vi "Flux_Capacitor_SoftFP.vi"(0 "reference in":refnum<class "Flux_Capacitor.lvclass">, 2 "Floating":bool, 5 "error in (no error)":errorcluster) -> (14 "reference out":refnum<class "Flux_Capacitor.lvclass">, 19 "error out":errorcluster)   [LabVIEW 2022 SP3, in "Flux_Capacitor.lvlib" / "Flux_Capacitor.lvclass"]
uses:
  Flux_Capacitor.lvclass
  Components/ViPER.lvlibp/ViPER.lvclass
  C:/Projects/Medulla/ViPER/Examples/Flux_Capacitor_Tester/Components/ViPER.lvlibp/ViPER.lvclass
panel:
  in  "Tab Control":enum32{"Flux", "Temp", "Time Circuit"}(tab)
  out "OK":bool
  in  "Flux Test":bool
  out "Temp table":i32(listbox)
  in  "Refresh Temps":bool
  in  "RTC":timestamp format="%<%X\n%x>T"
  in  "Refresh RTC":bool
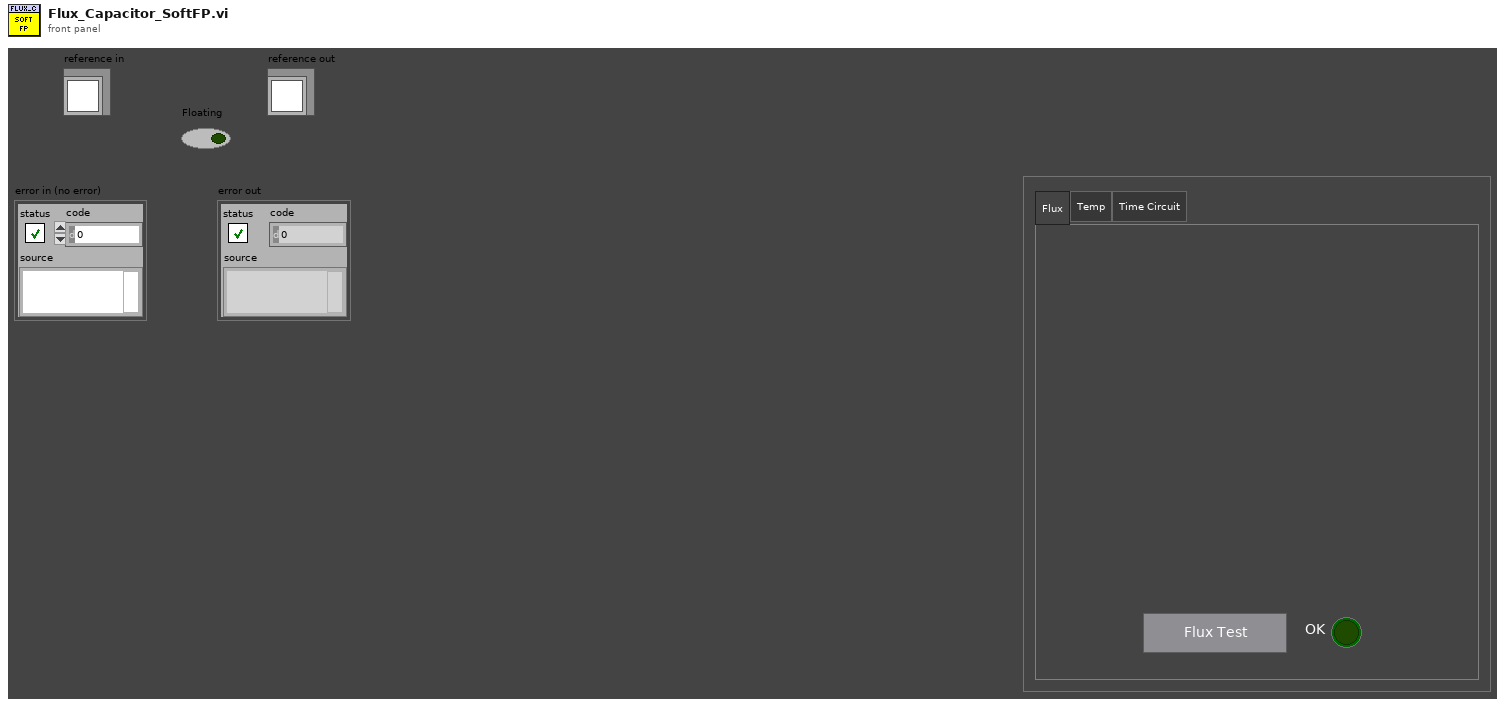
[diagram p1: front panel]
types:
  T1 = enum32{"Invalid", "Standard", "Closed", "Hidden", "Minimized", "Maximized"}
  T2 = typedef "Flux_Capacitor.lvlib/Flux_Capacitor.lvclass/ObjectAttributes.ctl" = cluster{"Config":T3, "T Sensors":T4[], "Temp_DegC":dbl[], "Temp_Raw":u64[], "RTC":timestamp, "Flux":bool, "Time":timestamp, "RTC_Live":timestamp}
  T3 = typedef "Flux_Capacitor.lvlib/Flux_Capacitor.lvclass/Config.ctl" = cluster{"default":string}
  T4 = typedef "Flux_Capacitor.lvlib/Flux_Capacitor.lvclass/TempSensor.ctl" = enum16{"1", "2", "3"}
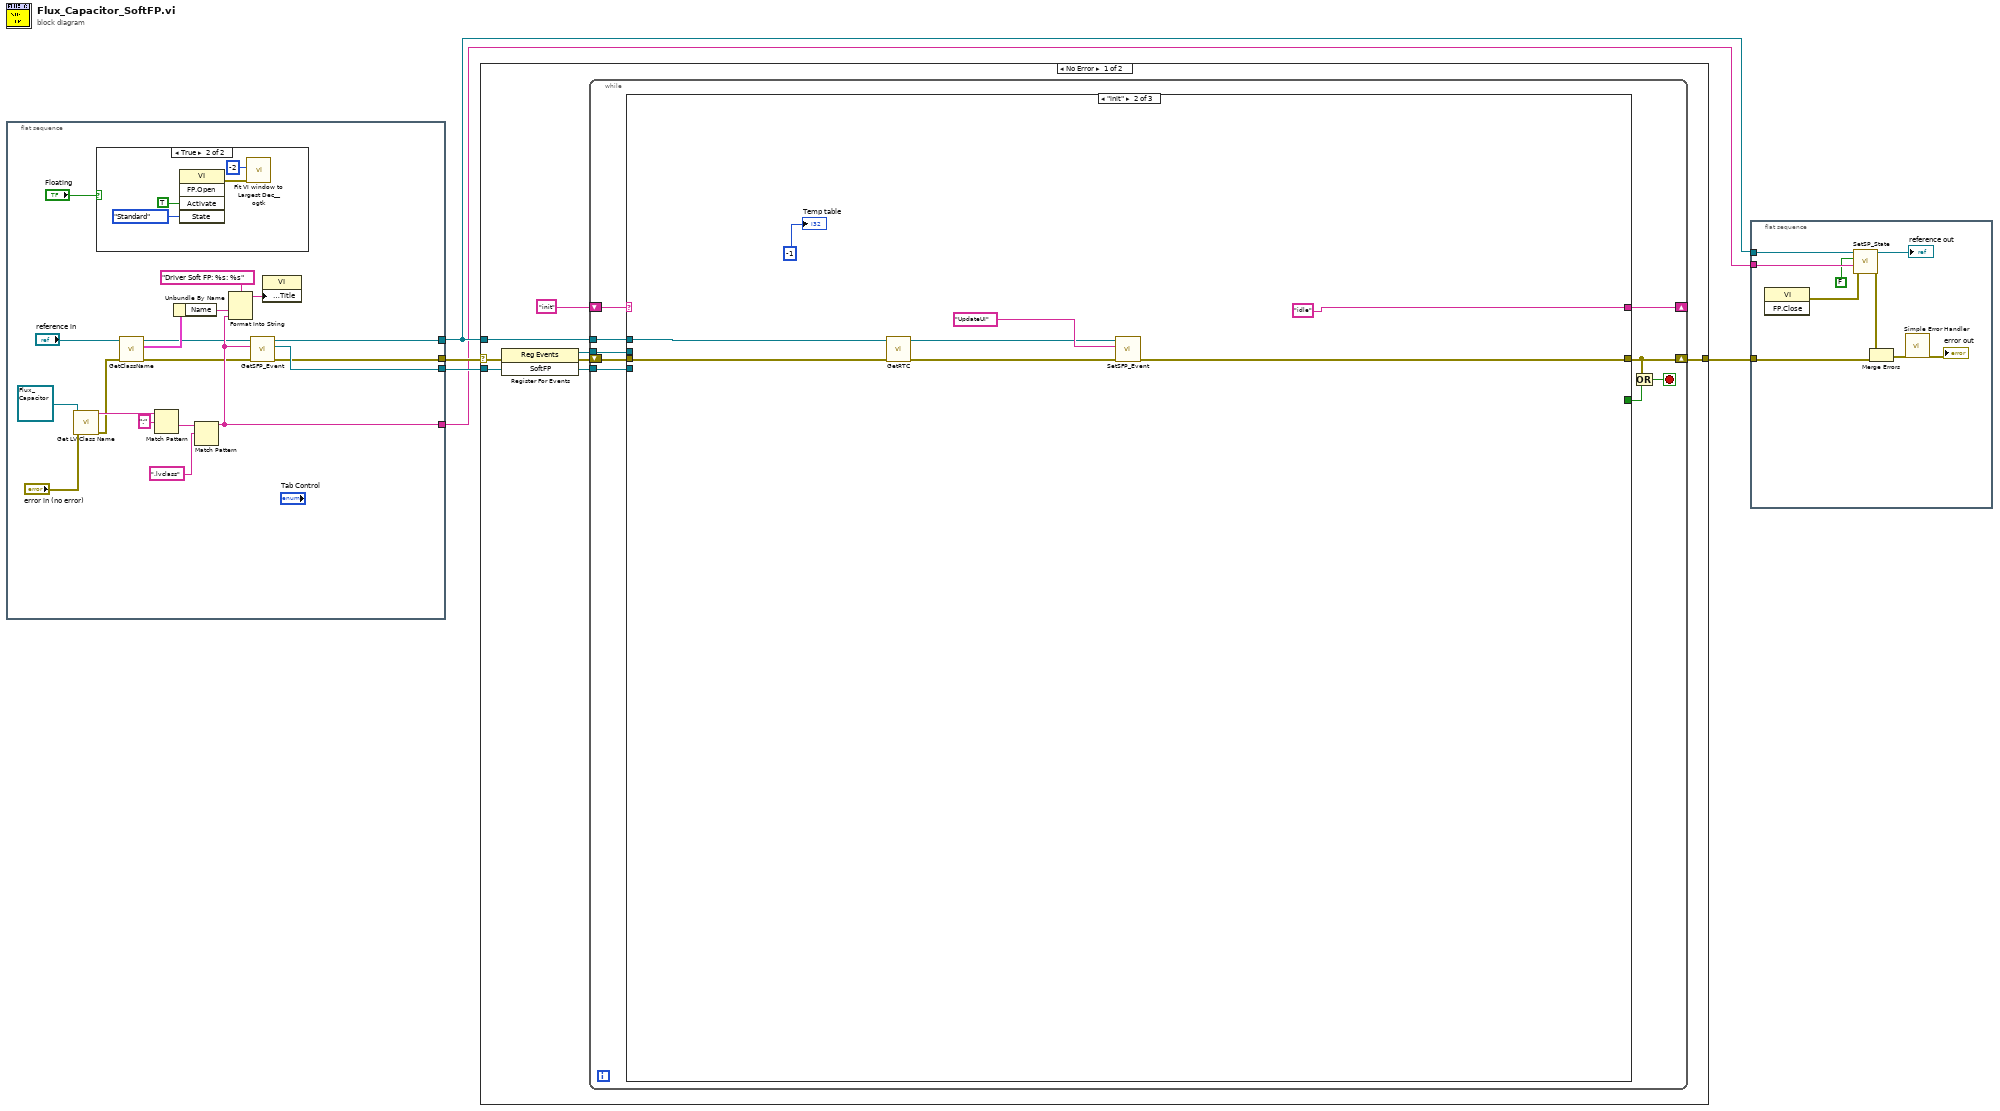
[diagram p0: block diagram]
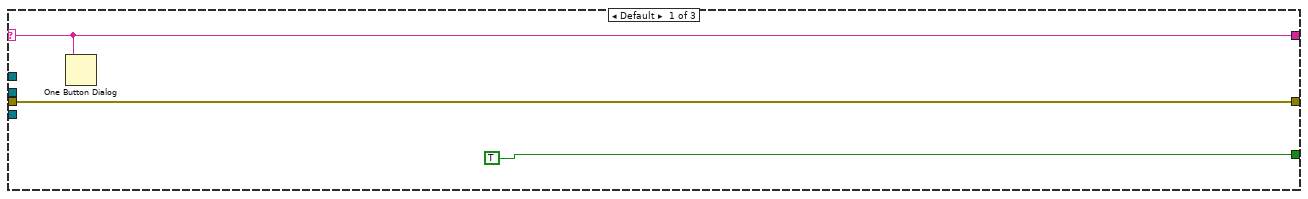
[diagram p3: hidden frame]
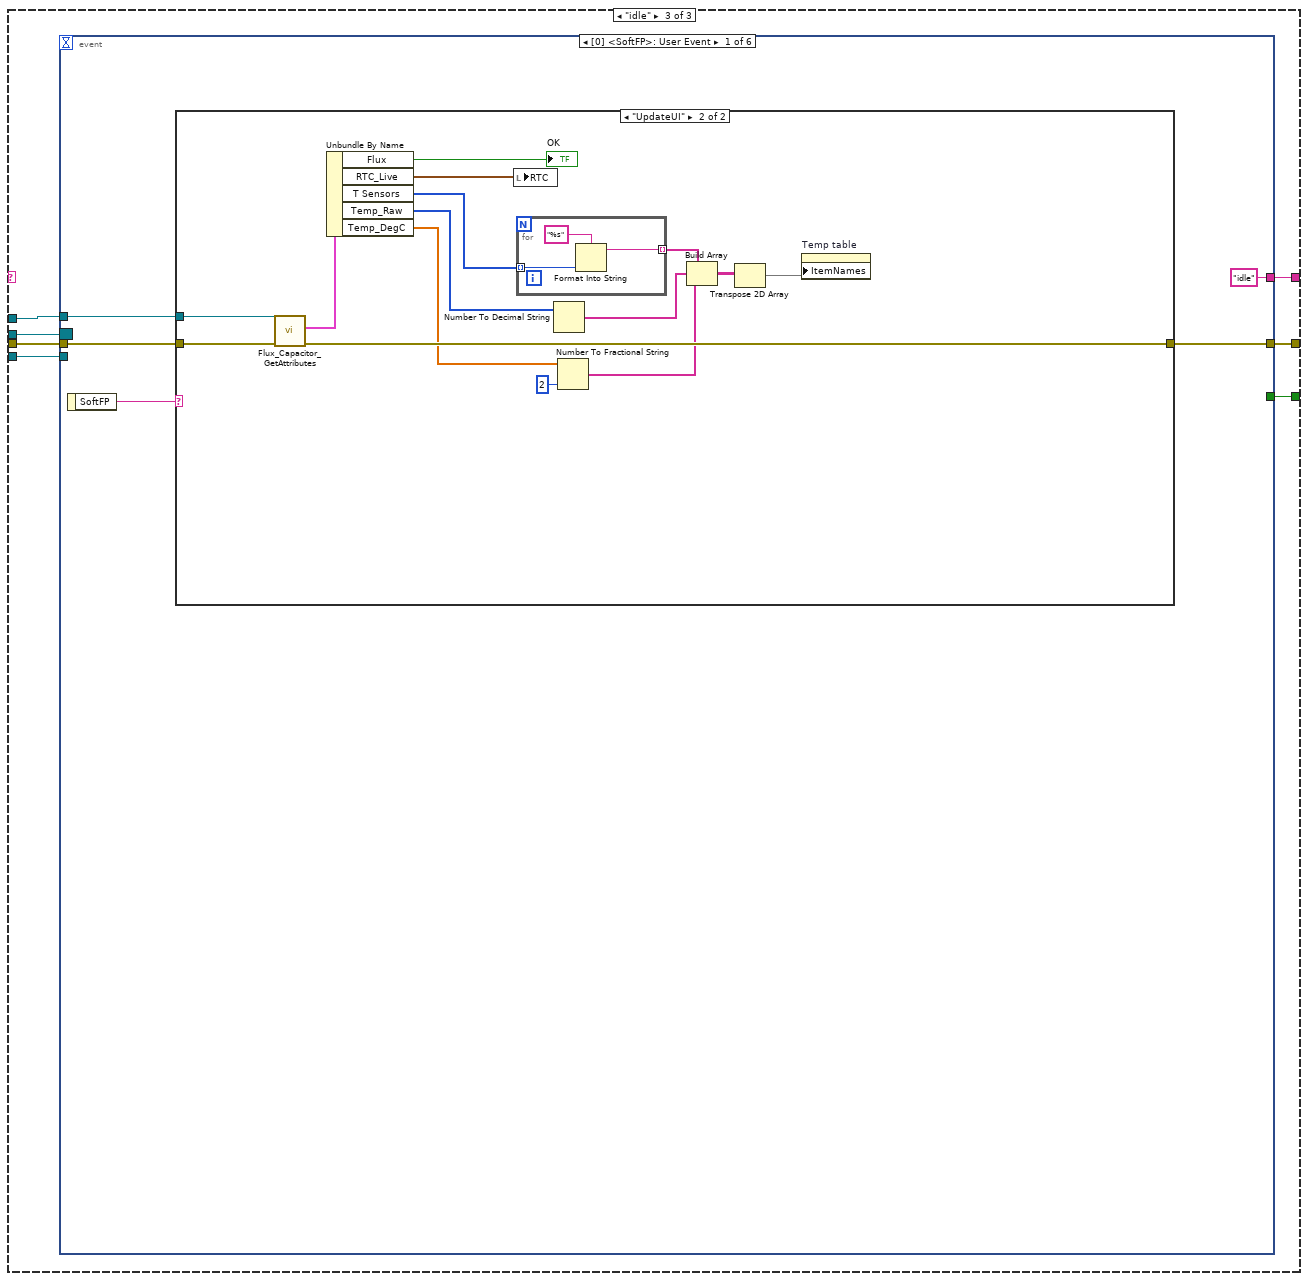
[diagram p4: hidden frame]
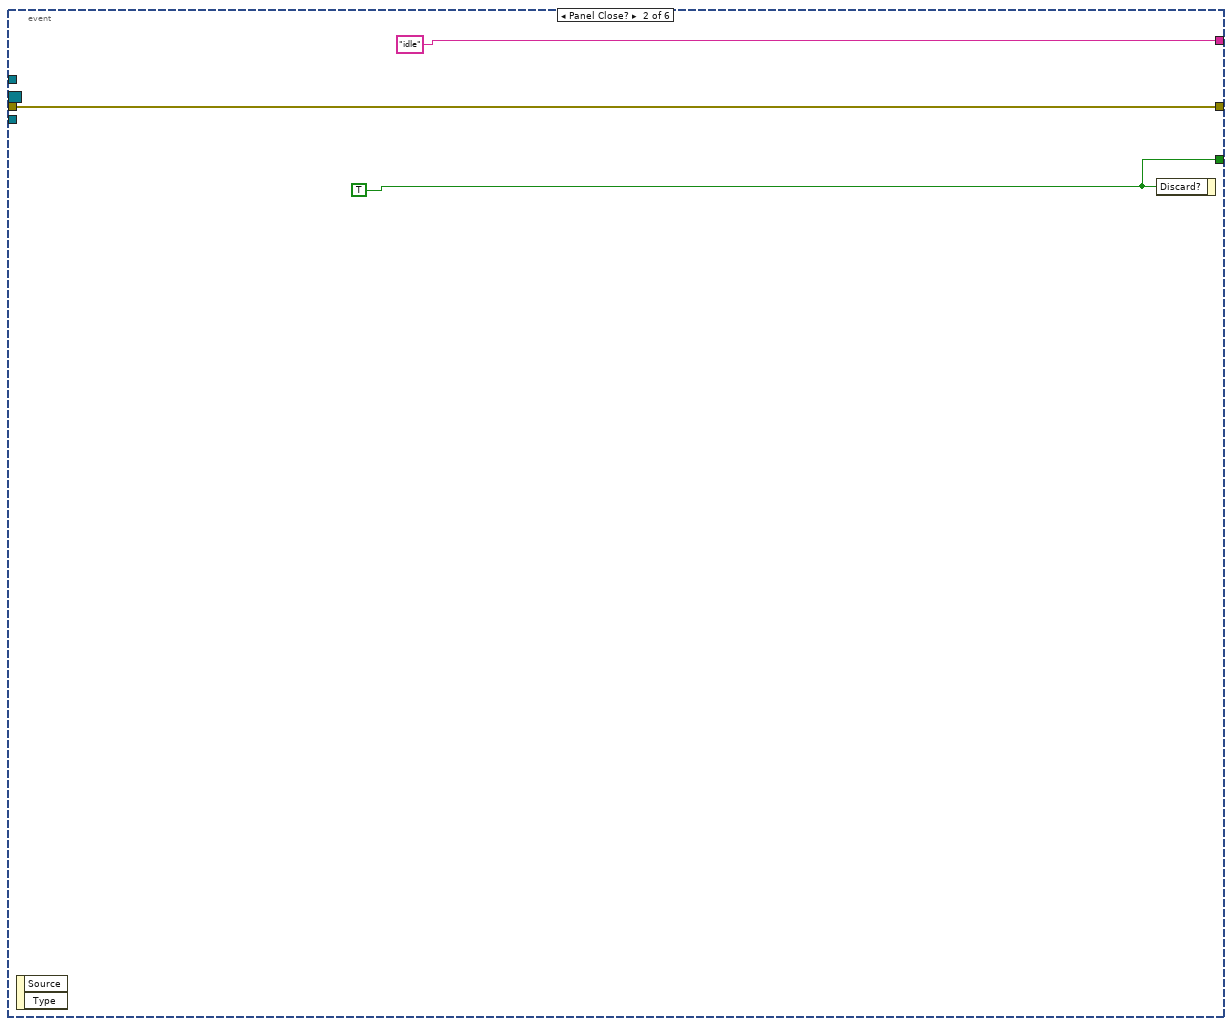
[diagram p6: hidden frame]
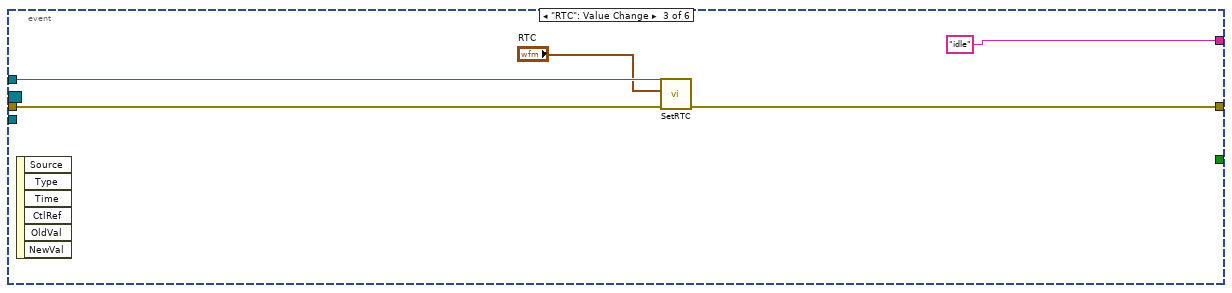
[diagram p7: hidden frame]
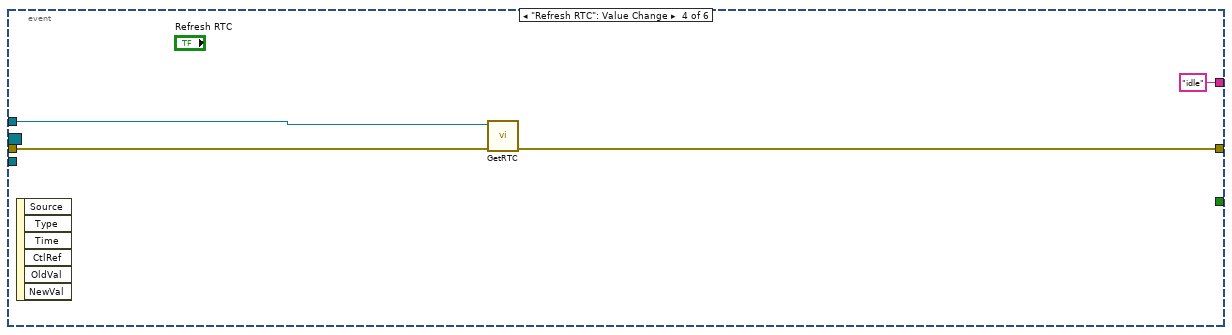
[diagram p8: hidden frame]
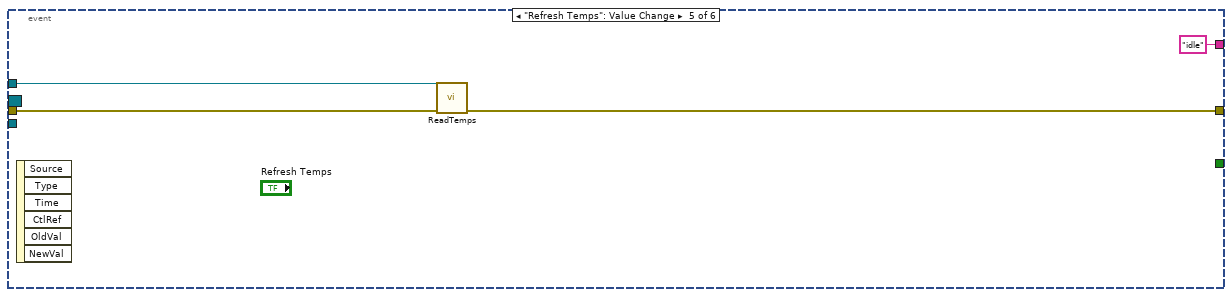
[diagram p9: hidden frame]
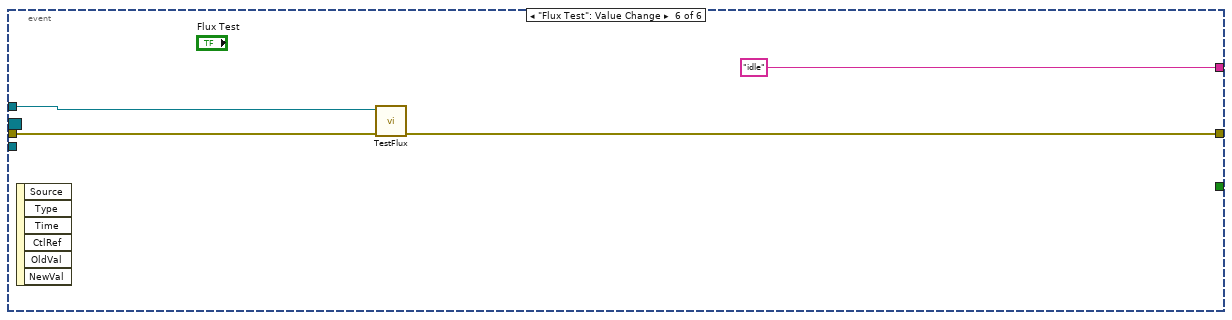
[diagram p10: hidden frame]
diagram:
  n1 = flat-sequence {
    tunnel: [w7] -> w5
    tunnel: [w6] -> w2
    tunnel: [w24] -> w3
    tunnel: [w14] -> w1
    frame #0 {
      n2 = call <vilib>:"Get LV Class Name.vi"("error in (no error)"="error in (no error)", "object"=refnum<class "Flux_Capacitor.lvclass"> refnum ("reference")) -> ("error out"=w13:errorcluster, "class name"=w19:string)  [unwired: 8 in]
      n3 = case shown="True" "Floating" {
        frame False {
        }
        frame True {
          n4 = invoke class="VI" method="FP.Open"("Activate"=TRUE ("Activate?"), "State"=T1."Standard") -> (error out=w25:errorcluster)  [unwired: 3 in, 4 out]
          n5 = call <userlib>:"Fit VI window to Largest Dec__ogtk.vi"("error in (no error)"=w25, "border spacing (2 px)"=-2) -> ()  [unwired: 4 in, 2 out]
        }
      }
      n6 = call "GetClassName.vi"("error in (no error)"=w13, "reference in"="reference in") -> ("error out"=w12:errorcluster, "Details"=w11:cluster{"Name":string, "Class":string}, "reference out"=w9:refnum<class "Flux_Capacitor.lvclass">)  [unwired: 7 in]
      n7 = Match Pattern(string=w19, regular expression=":") -> (after substring=w17:string)  [unwired: 1 in, 3 out]
      n8 = Unbundle By Name(w11) -> ("Name"=w21:string)
      n9 = Match Pattern(string=w17, regular expression=".lvclass") -> (before substring=w14:string)  [unwired: 1 in, 3 out]
      n10 = Format Into String(format string="Driver Soft FP: %s: %s", w21, w14) -> (resulting string=w23:string)  [unwired: 2 in, 1 out]
      n11 = call-dynamic "GetSFP_Event.vi"("error in (no error)"=w12, "Ancestor"=w14, "reference in"=w9) -> ("error out"=w7:errorcluster, "SoftFP"=w24:refnum<user-event>, "reference out"=w6:refnum<class "Flux_Capacitor.lvclass">)  [unwired: 6 in]
      n12 = property class="VI"("Front Panel.Title"=w23) -> ()  [unwired: 2 in, 2 out]
    }
  }
  n13 = case shown="No Error" w5 {
    selector: w5 -> [w34 w107]
    tunnel: [w30 w107] -> w4
    tunnel: w2 -> [w31 _]
    tunnel: w3 -> [w29 _]
    frame No Error {
      n14 = register-events(error in=w34, w29) -> (reference out=w35:refnum<event-registration>, error out=w33:errorcluster)  [unwired: 1 in]
      n15 = while {
        shift-right: [w41] -> w30
        shift-left: w33 -> [w44]
        tunnel: w35 -> [w43]
        tunnel: w31 -> [w42]
        shift-right: [w37] -> _
        shift-left: "init" -> [w38]
        tunnel: w29 -> [w36]
        stop <- w40 stop-if-true
        n16 = case shown="\"init\"" w38 {
          selector: w38 -> [w45 _ _]
          tunnel: w44 -> [w46 w50 w62]
          tunnel: w43 -> [_ _ w61]
          tunnel: w42 -> [_ w48 w60]
          tunnel: [w46 w53 w59] -> w41
          tunnel: [TRUE ("Discard?") _ w58] -> w39
          tunnel: [w45 "idle" w57] -> w37
          tunnel: w36 -> [_ _ w56]
          frame Default {
            n17 = One Button Dialog(message=w45) -> ()  [unwired: 1 in, 1 out]
          }
          frame "init" {
            n18 = call-dynamic "GetRTC.vi"("error in (no error)"=w50, "reference in"=w48) -> ("error out"=w51:errorcluster, "reference in"=w49:refnum<class "Flux_Capacitor.lvclass">)  [unwired: 6 in, 2 out]
            n19 = call-dynamic "SetSFP_Event.vi"("error in (no error)"=w51, "msg"="UpdateUI", "reference in"=w49) -> ("error out"=w53:errorcluster)  [unwired: 7 in, 1 out]
            "Temp table" <- -1 ("Pressure Table")
          }
          frame "idle" {
            n20 = event shown="[0] <SoftFP>: User Event" {
              selector: w61 -> [_ _ _ _ _ _]
              dyn-events: _ -> [_ _ _ _ _ _]
              timeout: _ -> [_ _ _ _ _ _]
              tunnel: w62 -> [w65 w89 w94 w97 w100 w106]
              tunnel: [w64 w89 w92 w98 w101 w104] -> w59
              tunnel: [_ w88 _ _ _ _] -> w58
              tunnel: w60 -> [w63 _ w93 w96 w99 w105]
              tunnel: ["idle" "idle" "idle" "idle" "idle" "idle"] -> w57
              tunnel: w56 -> [_ _ _ _ _ _]
              event User Event {
                n21 = event-data() -> ("SoftFP"=w66:string)  [unwired: 1 in]
                n22 = case shown="\"UpdateUI\"" w66 {
                  tunnel: w65 -> [w68 w82]
                  tunnel: [w68 w83] -> w64
                  tunnel: w63 -> [_ w81]
                  frame Default {
                  }
                  frame "UpdateUI" {
                    n23 = call "Flux_Capacitor_GetAttributes.vi"("error in (no error)"=w82, "reference in"=w81) -> ("error out"=w83:errorcluster, "Data"=w80:T2)  [unwired: 6 in, 2 out]
                    n24 = Unbundle By Name(w80) -> ("Flux"=→"OK":bool, "RTC_Live"=w69:timestamp, "T Sensors"=w78:T4[], "Temp_Raw"=w77:u64[], "Temp_DegC"=w76:dbl[])
                    n25 = local write "RTC"(w69) -> ()
                    n26 = for {
                      tunnel: w78 -> [w86] mode=indexing
                      tunnel: [w84] -> w74 mode=indexing
                      n27 = Format Into String(format string="%s", w86) -> (resulting string=w84:string)  [unwired: 2 in, 1 out]
                    }
                    n28 = Number To Decimal String(number=w77) -> (decimal integer string=w73:string[])  [unwired: 1 in]
                    n29 = Number To Fractional String(number=w76, precision (6)=i16 2) -> (F-format string=w72:string[])  [unwired: 2 in]
                    n30 = Build Array(w74, w73, w72) -> (w71:string[][])
                    n31 = Transpose 2D Array(2D array=w71) -> (transposed array=w70:string[][])
                    n32 = property on="Temp table" class="MCListbox (strict)"("ItemNames"=w70) -> ()  [unwired: 2 in, 2 out]
                  }
                }
              }
              event Panel Close? {
                w88 = TRUE ("Discard?")
                n33 = event-data() -> ()  [unwired: 1 in, 2 out]
                n34 = event-data("Discard?"=w88) -> ()  [unwired: 1 in, 1 out]
              }
              event "RTC": Value Change {
                n35 = event-data() -> ()  [unwired: 1 in, 6 out]
                n36 = call-dynamic "SetRTC.vi"("error in (no error)"=w94, "RTC"="RTC", "reference in"=w93) -> ("error out"=w92:errorcluster)  [unwired: 6 in, 2 out]
              }
              event "Refresh RTC": Value Change {
                n37 = event-data() -> ()  [unwired: 1 in, 6 out]
                n38 = call-dynamic "GetRTC.vi"("error in (no error)"=w97, "reference in"=w96) -> ("error out"=w98:errorcluster)  [unwired: 6 in, 3 out]
              }
              event "Refresh Temps": Value Change {
                n39 = event-data() -> ()  [unwired: 1 in, 6 out]
                n40 = call-dynamic "ReadTemps.vi"("error in (no error)"=w100, "reference in"=w99) -> ("error out"=w101:errorcluster)  [unwired: 6 in, 3 out]
              }
              event "Flux Test": Value Change {
                n41 = event-data() -> ()  [unwired: 1 in, 6 out]
                n42 = call-dynamic "TestFlux.vi"("error in (no error)"=w106, "reference in"=w105) -> ("error out"=w104:errorcluster)  [unwired: 7 in, 2 out]
              }
            }
          }
        }
        n43 = Or(x=w41, y=w39) -> (x .or. y?=w40:bool)
      }
    }
    frame Error {
    }
  }
  n44 = flat-sequence {
    tunnel: w4 -> [w114]
    tunnel: w2 -> [w109]
    tunnel: w1 -> [w111]
    frame #0 {
      n45 = invoke class="VI" method="FP.Close"() -> (error out=w113:errorcluster)  [unwired: 3 in, 2 out]
      n46 = call "SetSP_State.vi"("error in (no error)"=w113, "Ancestor"=w111, "SP Open"=FALSE, "reference in"=w109) -> ("error out"=w112:errorcluster, "reference out"=→"reference out":refnum<class "Flux_Capacitor.lvclass">)  [unwired: 6 in]
      n47 = Merge Errors(w112, w114) -> (w116:errorcluster)
      n48 = call <vilib>:"Simple Error Handler.vi"("error in (no error)"=w116) -> ("error out"=→"error out":errorcluster)  [unwired: 4 in, 4 out]
    }
  }
